vi "Send Start Pattern.vi"(7 "Message Priority (Normal)":T1=enum."Normal", 8 "error in (no error)":errorcluster, 9 "Timeout":i32, 10 "Start Address":i32, 11 "Message Enqueuer":refnum<class "Message Enqueuer.lvclass">) -> (0 "error out":errorcluster, 3 "Message Enqueuer out":refnum<class "Message Enqueuer.lvclass">)   [LabVIEW 2015, in "CS++PPG.lvlib" / "Start Pattern Msg.lvclass"]
doc: "Sends the <B>CS++PPG.lvlib:Start Pattern Msg.lvclass</B> message.\n\n<B>CS++PPG.lvlib:CS++PPG.lvclass:Start Pattern.vi</B> Description:\n\nThis VI starts the execution of the pattern (depending on the settings this could mean that the device first waits for an hardware trigger)."
uses:
  Start Pattern Msg.lvclass
  <vilib>/ActorFramework/Message Enqueuer/Message Enqueuer.lvclass
  <vilib>/ActorFramework/Message Enqueuer/Message Priority.ctl
  Start Pattern Msg.lvclass/Start Pattern Msg.ctl
  <vilib>/ActorFramework/Message Enqueuer/Message Enqueuer.lvclass/Message Enqueuer.ctl
  <vilib>/ActorFramework/Message Priority Queue/Priority Enqueue.vi
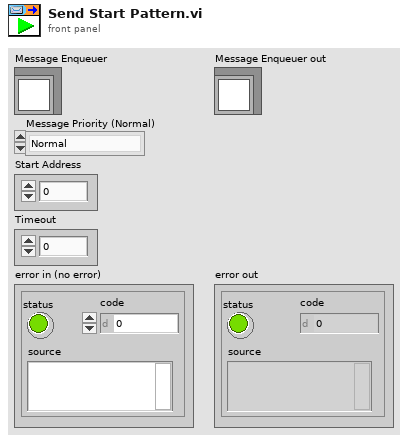
[diagram p1: front panel]
types:
  T1 = typedef "Actor Framework.lvlib/Message Enqueuer.lvclass/Message Priority.ctl" = enum16{"Low", "Normal", "High"}
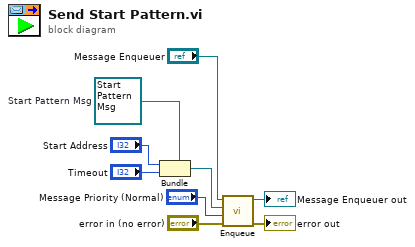
[diagram p0: block diagram]
diagram:
  w3 = refnum<class "Start Pattern Msg.lvclass"> refnum  # Start Pattern Msg
  n1 = Bundle(cluster=w3, "Start Address", "Timeout") -> (w6:refnum<class "Start Pattern Msg.lvclass">)
  n2 = call <vilib>:"Enqueue.vi"("error in (no error)"="error in (no error)", "Message Priority (Normal)"="Message Priority (Normal)", "Message"=w6, "Message Enqueuer in"="Message Enqueuer") -> ("error out"=→"error out":errorcluster, "Message Enqueuer out"=→"Message Enqueuer out":refnum<class "Message Enqueuer.lvclass">)  [unwired: 6 in]
